vi "GetTreeStack.vi"(8 "error in":errorcluster, 11 "node in":refnum<data-value>) -> (0 "error out":errorcluster, 3 "parents":refnum<data-value>[](array[refnum]))   [LabVIEW 2013, in "NISE_CEF_Node.lvclass"]
uses:
  NISE_CEF_Node.lvclass
  NISE_CEF_Node.lvclass/NISE_CEF_Node.ctl
  ReadParent.vi
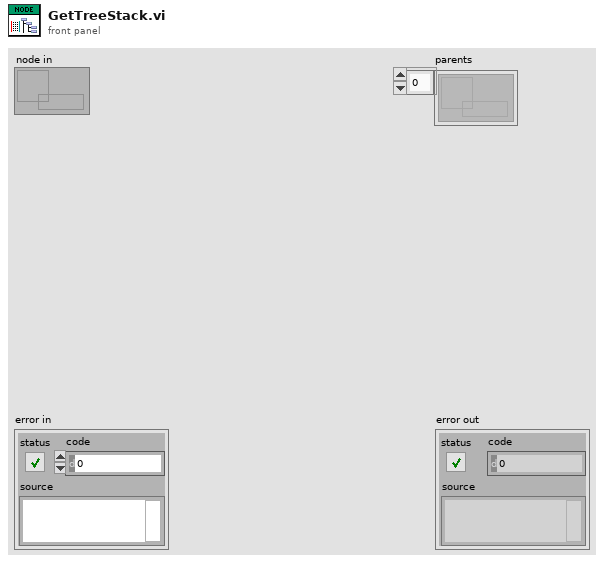
[diagram p1: front panel]
types:
  T1 = typedef "NISE_CEF_Node.lvclass/NodeRef.ctl" = refnum<data-value>
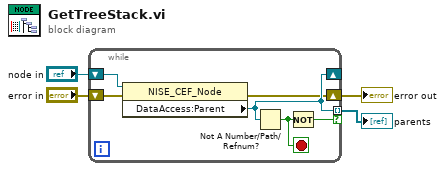
[diagram p0: block diagram]
diagram:
  n1 = while {
    shift-right: [w6] -> _
    shift-left: "node in" -> [w9]
    tunnel: [w6] -> w2 mode=indexing if=w7
    shift-right: [w5] -> w1
    shift-left: "error in" -> [w10]
    stop <- w8 stop-if-true
    n2 = property class="NISE_CEF_Node"(reference=w9, error in=w10) -> (error out=w5:errorcluster, "DataAccess:Parent"=w6:T1)  [unwired: 1 out]
    n3 = Not A Number/Path/Refnum?(number/path/refnum=w6) -> (NaN/Path/Refnum?=w8:bool)
    n4 = Not(x=w8) -> (.not. x?=w7:bool)
  }
  "error out" <- w1
  "parents" <- w2
